vi "4200_measurement_option.vi"() -> ()   [LabVIEW 2013]
uses:
  <vilib>/Instr/_visa.llb/VISA Event Mechanism.ctl
  <vilib>/Instr/_visa.llb/Select Event Type.ctl
panel:
  in  "Measurement mode":enum16{"Resistor", "Transistor", "Diode"}(ring)
  out "XY Graph":cluster{dbl[], dbl[]}(graph)
  out "Current (A)    Voltage (V)":dbl[][](array[numeric]) caption="appended array"
  out "Resistance (Ohm)":dbl
  out "Waveform Chart 3":cluster{dbl}(graph)
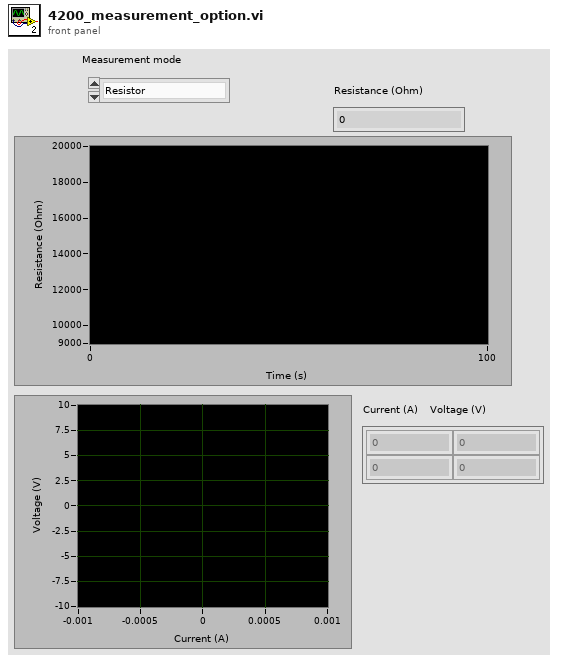
[diagram p1: front panel]
types:
  T1 = typedef "Select Event Type.ctl" = u32
  T2 = typedef "VISA Event Mechanism.ctl" = u16
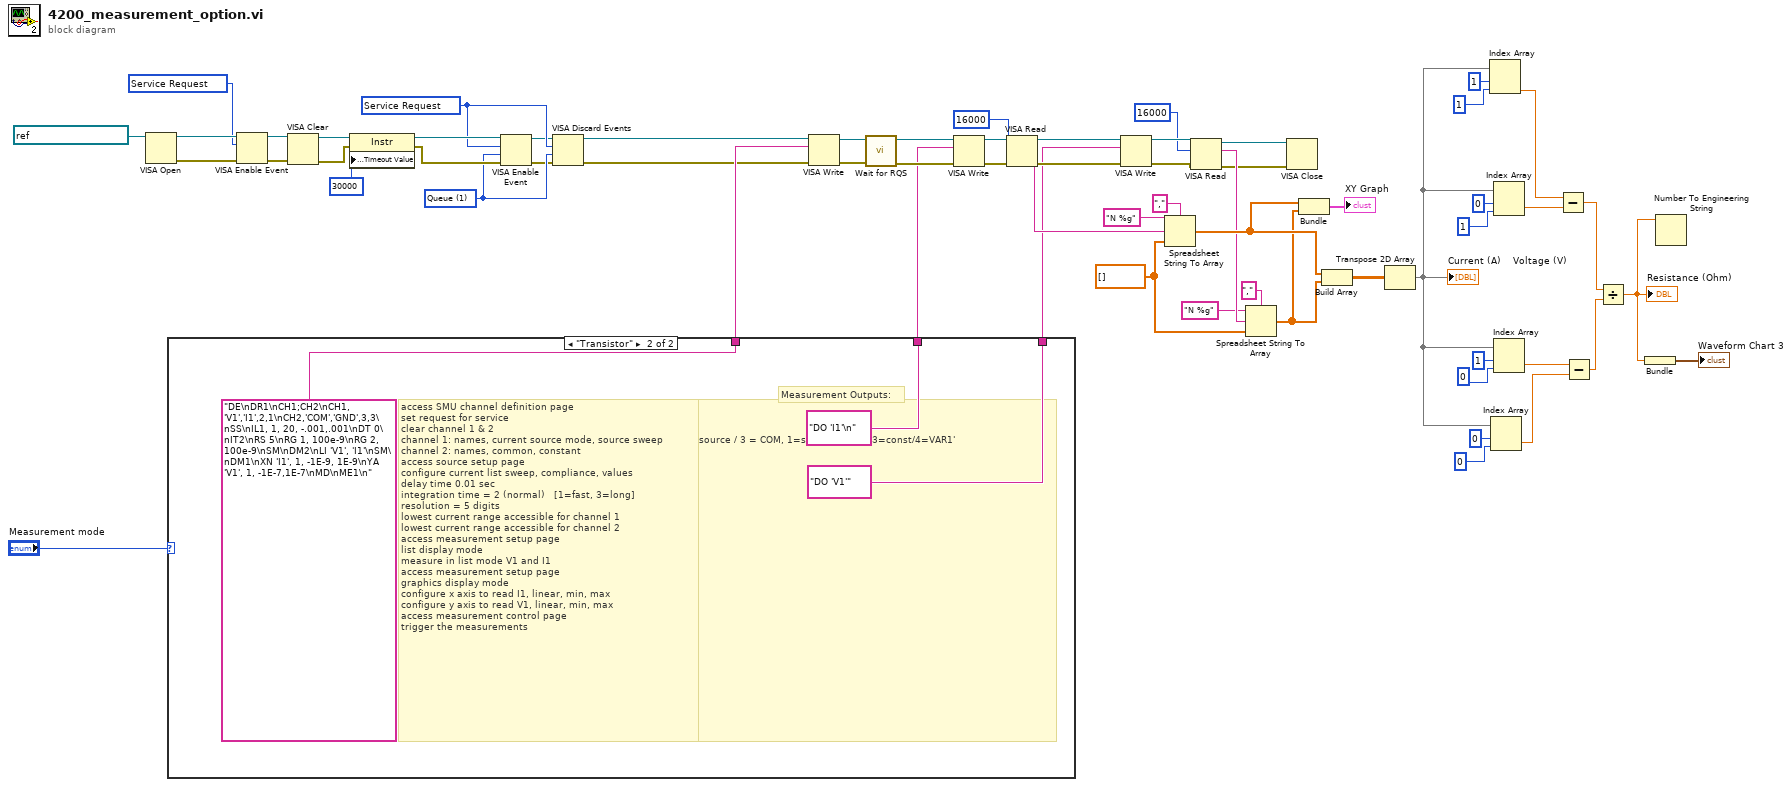
[diagram p0: block diagram]
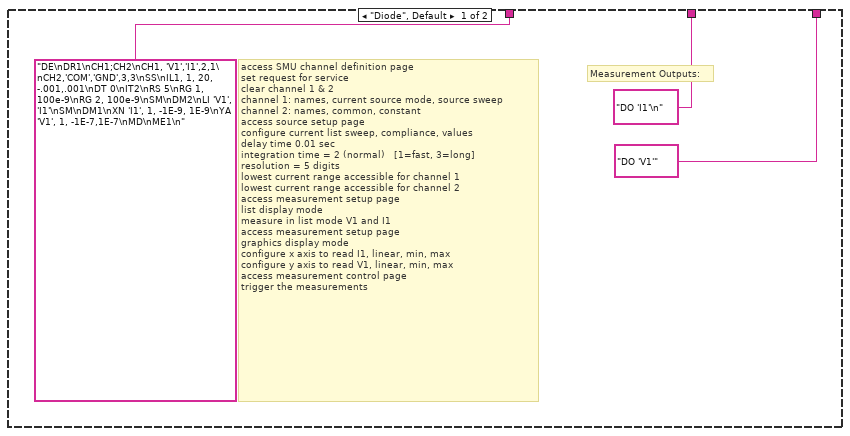
[diagram p2: hidden frame]
diagram:
  w40 = dbl[] []
  w60 = T1 1073684491 items=["Service Request"=1073684491, "Trigger"=3221168138, "Clear"=1073684493, "VXI Signal"=1073684512, "VXI/VME Interrupt"=3221168161, "VXI/VME Sysfail"=1073684509, "VXI/VME Sysreset"=1073684510, "GPIB CIC"=1073684498, "GPIB Talk"=1073684499, "GPIB Listen"=1073684500, "PXI Interrupt"=1073684514, "Serial Break"=1073684515, "Serial TermChar"=1073684516, "Serial CTS"=1073684521, "Serial DSR"=1073684522, "Serial DCD"=1073684524, "Serial RI"=1073684526, "Serial Character"=1073684533, "USB Interrupt"=1073684535, "All Enabled"=1073709055] ("Event Type")
  w53 = T2 1 items=["Queue"=1] ("Mechanism Type")
  w52 = T1 1073684491 items=["Service Request"=1073684491, "Trigger"=3221168138, "Clear"=1073684493, "VXI Signal"=1073684512, "VXI/VME Interrupt"=3221168161, "VXI/VME Sysfail"=1073684509, "VXI/VME Sysreset"=1073684510, "GPIB CIC"=1073684498, "GPIB Talk"=1073684499, "GPIB Listen"=1073684500, "PXI Interrupt"=1073684514, "Serial Break"=1073684515, "Serial TermChar"=1073684516, "Serial CTS"=1073684521, "Serial DSR"=1073684522, "Serial DCD"=1073684524, "Serial RI"=1073684526, "Serial Character"=1073684533, "USB Interrupt"=1073684535, "All Enabled"=1073709055] ("Event Type")
  n1 = VISA Open(VISA resource name=refnum<visa-resource-name> "GPIB0::17::INSTR") -> (VISA resource name=w62:refnum<visa-resource-name>, error out=w63:errorcluster)  [unwired: 1 in, 3 out]
  n2 = case shown="\"Transistor\"" "Measurement mode" {
    tunnel: ["DE\nDR1\nCH1;CH2\nCH1, 'V1','I1',2,1\nCH2,'COM','GND',3,3\nSS\nIL1, 1, 20, -.001,.001\nDT 0\nIT2\nRS 5\nRG 1, 100e-9\nRG 2, 100e-9\nSM\nDM2\nLI 'V1', 'I1'\nSM\nDM1\nXN 'I1', 1, -1E-9, 1E-9\nYA 'V1', 1, -1E-7,1E-7\nMD\nME1\n" ("write buffer") "DE\nDR1\nCH1;CH2\nCH1, 'V1','I1',2,1\nCH2,'COM','GND',3,3\nSS\nIL1, 1, 20, -.001,.001\nDT 0\nIT2\nRS 5\nRG 1, 100e-9\nRG 2, 100e-9\nSM\nDM2\nLI 'V1', 'I1'\nSM\nDM1\nXN 'I1', 1, -1E-9, 1E-9\nYA 'V1', 1, -1E-7,1E-7\nMD\nME1\n" ("write buffer")] -> w14
    tunnel: ["DO 'I1'\n" "DO 'I1'\n"] -> w2
    tunnel: ["DO 'V1'" ("write buffer") "DO 'V1'" ("write buffer")] -> w1
    frame "Diode", Default {
      # "Measurement Outputs:"
      # "access SMU channel definition page\nset request for service\nclear channel 1 & 2\nchannel 1: names, current source mode, source sweep\nchannel 2: names, common, constant\naccess source setup page\nconfigure current list sweep, compliance, values\ndelay time 0.01 sec\nintegration time = 2 (normal)   [1=fast, 3=long]\nresolution = 5 digits\nlowest current range accessible for channel 1\nlowest current range accessible for channel 2\naccess measurement setup page\nlist display mode\nmeasure in list mode V1 and I1\naccess measurement setup page\ngraphics display mode\nconfigure x axis to read I1, linear, min, max\nconfigure y axis to read V1, linear, min, max\naccess measurement control page\ntrigger the measurements"
    }
    frame "Transistor" {
      # "access SMU channel definition page\nset request for service\nclear channel 1 & 2\nchannel 1, voltage name, current name, 1 = V source / 2 = I source / 3 = COM, 1=sweep/2=step/3=const/4=VAR1' \n\n\n\ncurrent source mode, source sweep\nchannel 2: names, common, constant\naccess source setup page\nconfigure current list sweep, compliance, values\ndelay time 0.01 sec\nintegration time = 2 (normal)   [1=fast, 3=long]\nresolution = 5 digits\nlowest current range accessible for channel 1\nlowest current range accessible for channel 2\naccess measurement setup page\nlist display mode\nmeasure in list mode V1 and I1\naccess measurement setup page\ngraphics display mode\nconfigure x axis to read I1, linear, min, max\nconfigure y axis to read V1, linear, min, max\naccess measurement control page\ntrigger the measurements"
      # "Measurement Outputs:"
      # "access SMU channel definition page\nset request for service\nclear channel 1 & 2\nchannel 1: names, current source mode, source sweep\nchannel 2: names, common, constant\naccess source setup page\nconfigure current list sweep, compliance, values\ndelay time 0.01 sec\nintegration time = 2 (normal)   [1=fast, 3=long]\nresolution = 5 digits\nlowest current range accessible for channel 1\nlowest current range accessible for channel 2\naccess measurement setup page\nlist display mode\nmeasure in list mode V1 and I1\naccess measurement setup page\ngraphics display mode\nconfigure x axis to read I1, linear, min, max\nconfigure y axis to read V1, linear, min, max\naccess measurement control page\ntrigger the measurements"
    }
  }
  n3 = VISA Enable Event(8:w63, 10:w60, 11:w62) -> (0:w59:errorcluster, 3:w58:refnum<visa-resource-name>)  [unwired: 1 out]
  n4 = VISA Clear(VISA resource name=w58, error in (no error)=w59) -> (VISA resource name out=w54:refnum<visa-resource-name>, error out=w55:errorcluster)
  n5 = property class="Instr"(reference=w54, error in=w55, "General Settings:Timeout Value"=u32 30000) -> (reference out=w56:refnum<visa-resource-name>, error out=w57:errorcluster)
  n6 = VISA Enable Event(8:w57, 9:w53, 10:w52, 11:w56) -> (0:w51:errorcluster, 3:w50:refnum<visa-resource-name>)
  n7 = VISA Discard Events(8:w51, 9:w53, 10:w52, 11:w50) -> (0:w6:errorcluster, 3:w7:refnum<visa-resource-name>)
  n8 = VISA Write(VISA resource name=w7, write buffer=w14, error in (no error)=w6) -> (VISA resource name out=w15:refnum<visa-resource-name>, error out=w16:errorcluster)  [unwired: 1 out]
  n9 = call <vilib>:"Wait for RQS.vi"("error in (no error)"=w16, "VISA resource name"=w15) -> ("error out"=w12:errorcluster, "VISA resource name out"=w13:refnum<visa-resource-name>)  [unwired: 1 in, 7 out]
  n10 = VISA Write(VISA resource name=w13, write buffer=w2, error in (no error)=w12) -> (VISA resource name out=w48:refnum<visa-resource-name>, error out=w45:errorcluster)  [unwired: 1 out]
  n11 = VISA Read(VISA resource name=w48, byte count=u32 16000, error in (no error)=w45) -> (VISA resource name out=w47:refnum<visa-resource-name>, read buffer=w33:string, error out=w44:errorcluster)  [unwired: 1 out]
  n12 = VISA Write(VISA resource name=w47, write buffer=w1, error in (no error)=w44) -> (VISA resource name out=w42:refnum<visa-resource-name>, error out=w43:errorcluster)  [unwired: 1 out]
  n13 = Spreadsheet String To Array(delimiter (Tab)=",", format string="N %g", spreadsheet string=w33, array type (2D Dbl)=w40) -> (array=w37:dbl[])
  n14 = VISA Read(VISA resource name=w42, byte count=u32 16000, error in (no error)=w43) -> (VISA resource name out=w5:refnum<visa-resource-name>, read buffer=w32:string, error out=w4:errorcluster)  [unwired: 1 out]
  n15 = Spreadsheet String To Array(delimiter (Tab)=",", format string="N %g", spreadsheet string=w32, array type (2D Dbl)=w40) -> (array=w36:dbl[])
  n16 = VISA Close(VISA resource name=w5, error in (no error)=w4) -> ()  [unwired: 1 out]
  n17 = Bundle(w37, w36) -> (→"XY Graph":cluster{dbl[], dbl[]})  [unwired: 1 in]
  n18 = Build Array(w37, w36) -> (w34:dbl[][])
  n19 = Transpose 2D Array(2D array=w34) -> (transposed array=w19:dbl[][])
  "Current (A)    Voltage (V)" <- w19
  n20 = Index Array(array=w19, index (row)=1, index (col)=1 ("index (row)")) -> (element=w21:dbl)
  n21 = Index Array(array=w19, index (row)=0, index (col)=0 ("index (row)")) -> (element=w22:dbl)
  n22 = Index Array(array=w19, index (row)=0, index (col)=1 ("index (row)")) -> (element=w20:dbl)
  n23 = Index Array(array=w19, index (row)=1, index (col)=0 ("index (row)")) -> (element=w23:dbl)
  n24 = Subtract(x=w21, y=w20) -> (x-y=w17:dbl)
  n25 = Subtract(x=w23, y=w22) -> (x-y=w18:dbl)
  n26 = Divide(x=w17, y=w18) -> (x/y=w8:dbl)
  "Resistance (Ohm)" <- w8
  n27 = Bundle(w8) -> (→"Waveform Chart 3":cluster{dbl})  [unwired: 1 in]
  n28 = Number To Engineering String(4:w8) -> ()  [unwired: 3 in, 1 out]
